vi "Create Connection with CD.vi"(8 "error in (no error)":errorcluster, 10 "IP Address":string, 11 "TCP Service":string) -> (0 "error out":errorcluster, 3 "Connection Info Out":T1)   [LabVIEW 2015, in "PID Control Host API.lvlib"]
uses:
  PID Control Host API.lvlib
  <vilib>/NI/STM/compatibility/stm_TCP Connection Info.ctl
  <vilib>/NI/STM/compatibility/stm_MetaDataElement.ctl
  <vilib>/NI/STM/compatibility/stm_TCP Write Options.ctl
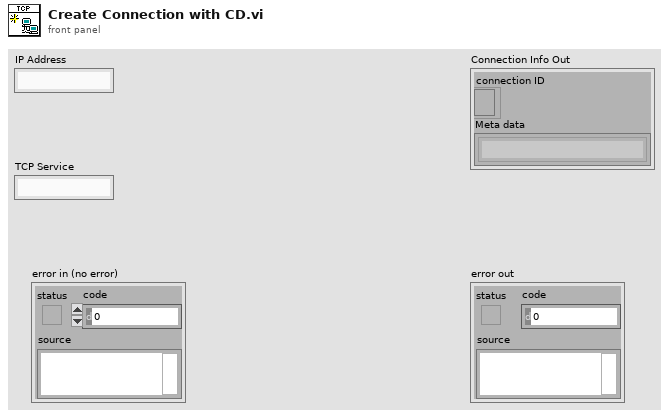
[diagram p1: front panel]
types:
  T1 = typedef "stm_TCP Connection Info.ctl" = cluster{"connection ID":refnum<k5>, "Meta data":T2[]}
  T2 = typedef "stm_MetaDataElement.ctl" = string
  T3 = typedef "stm_TCP Write Options.ctl" = cluster{"Ignore Timeout Error":bool, "timeout ms (1000)":i32}
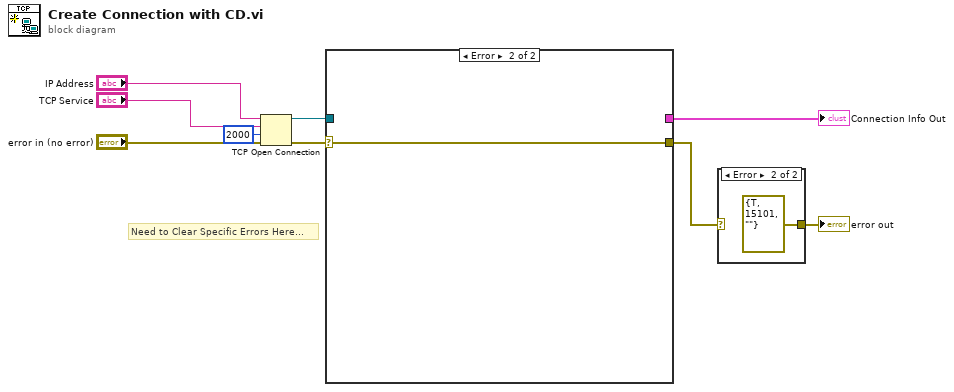
[diagram p0: block diagram]
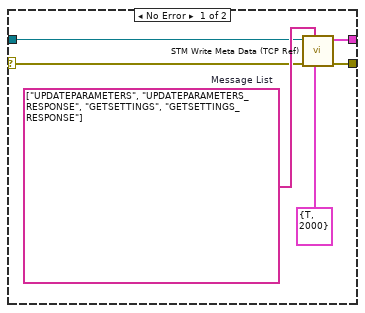
[diagram p3: hidden frame]
diagram:
  # "Need to Clear Specific Errors Here..."
  n1 = TCP Open Connection(address="IP Address", remote port or service name="TCP Service", timeout ms (60000)=2000, error in (no error)="error in (no error)") -> (connection ID=w9:refnum<k5>, error out=w8:errorcluster)  [unwired: 1 in]
  n2 = case shown="Error" w8 {
    selector: w8 -> [w11 w16]
    tunnel: w9 -> [w14 _]
    tunnel: [w13 w16] -> w2
    tunnel: [w12 _] -> w6
    frame No Error {
      w15 = string[] ["UPDATEPARAMETERS", "UPDATEPARAMETERS_RESPONSE", "GETSETTINGS", "GETSETTINGS_RESPONSE"]  # Message List
      n3 = call <vilib>:"STM Write Meta Data (TCP Ref).vi"("Options"=T3 {"Ignore Timeout Error"=TRUE, "timeout ms (1000)"=2000}, "Meta data"=w15, "error in"=w11, "connection ID"=w14) -> ("error out"=w13:errorcluster, "Connection Info Out"=w12:T1)  [unwired: 6 in]
    }
    frame Error {
    }
  }
  "Connection Info Out" <- w6
  n4 = case shown="Error" w2 {
    selector: w2 -> [w17 _]
    tunnel: [w17 errorcluster {"status"=TRUE, "code"=15101, "source"=""} ("error IO")] -> w1
    frame No Error {
    }
    frame Error {
    }
  }
  "error out" <- w1
